vi "IS Open Connection.vi"(8 "error in (no error)":errorcluster, 11 "Access Key":string) -> (0 "error out":errorcluster, 3 "IS Session":T1)   [LabVIEW 2013]
doc: "This VI opens a new HTTP Request with the Initial State API. You provide your Initial State Access Key and receive an active Initial State session with proper headers already set."
uses:
  <vilib>/httpClient/LabVIEWHTTPClient.lvlib
  <vilib>/httpClient/ClientHandle.ctl
  Controls/IS Session.ctl
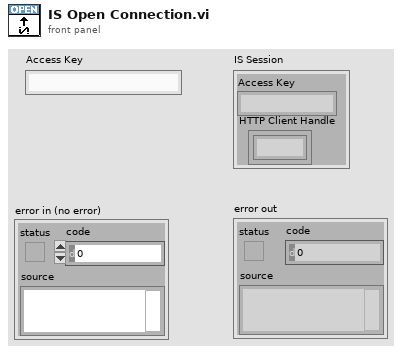
[diagram p1: front panel]
types:
  T1 = typedef "IS Session.ctl" = cluster{"Access Key":string, "HTTP Client Handle":T2}
  T2 = typedef "LabVIEWHTTPClient.lvlib/ClientHandle.ctl" = refnum<k1>
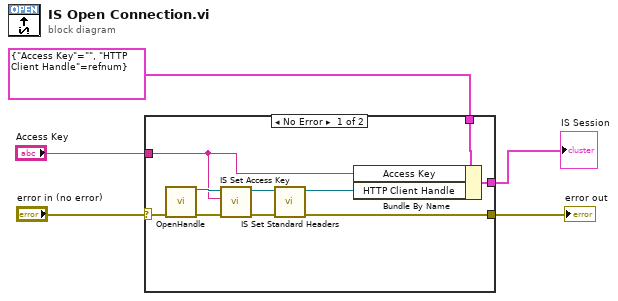
[diagram p0: block diagram]
diagram:
  n1 = case shown="No Error" "error in (no error)" {
    selector: "error in (no error)" -> [w15 w17]
    tunnel: [w6 w17] -> w5
    tunnel: "Access Key" -> [w10 _]
    tunnel: [w14 w16] -> w2
    tunnel: T1 {"Access Key"="", "HTTP Client Handle"=refnum} ("IS Session") -> [w13 w16]
    frame No Error {
      n2 = call <vilib>:"OpenHandle.vi"("error in (no error)"=w15) -> ("client handle out"=w12:T2, "error out"=w11:errorcluster)  [unwired: 13 in]
      n3 = call "IS Set Access Key.vi"("HTTP Client Handle in"=w12, "Access Key"=w10, "error in (no error)"=w11) -> ("HTTP Client Handle out"=w9:T2, "error out"=w8:errorcluster)  [unwired: 6 in]
      n4 = call "IS Set Standard Headers.vi"("error in (no error)"=w8, "client handle"=w9) -> ("error out"=w6:errorcluster, "client handle out"=w7:T2)  [unwired: 8 in]
      n5 = Bundle By Name(cluster=w13, "Access Key"=w10, "HTTP Client Handle"=w7) -> (w14:T1)
    }
    frame Error {
    }
  }
  "error out" <- w5
  "IS Session" <- w2
